vi "WPI_DashboardSeparate Tagged UDP Data.vi"(11 "String":string) -> (3 "Tagged Array":cluster{u8, u8, "unsigned byte array":u8[]}[](array[cluster]))   [LabVIEW 2017]
panel:
  out "size(s)":i32
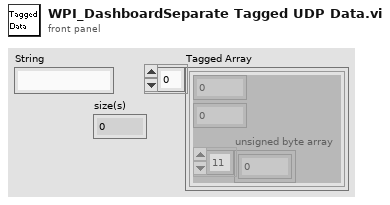
[diagram p1: front panel]
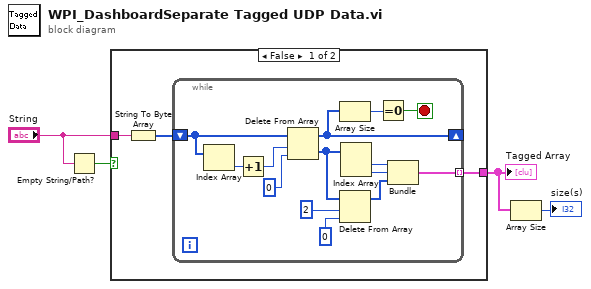
[diagram p0: block diagram]
diagram:
  n1 = Empty String/Path?(string/path="String") -> (empty?=w3:bool)
  n2 = case shown="False" w3 {
    tunnel: "String" -> [w7 _]
    tunnel: [w5 _] -> w2
    frame False {
      n3 = String To Byte Array(string=w7) -> (unsigned byte array=w6:u8[])
      n4 = while {
        shift-right: [w9] -> _
        shift-left: w6 -> [w21]
        tunnel: [w8] -> w5 mode=indexing
        stop <- w11 stop-if-true
        n5 = Index Array(array=w21) -> (element=w20:u8)  [unwired: 1 in]
        n6 = Increment(x=w20) -> (x+1=w19:u8)
        n7 = Delete From Array(array=w21, length=w19, index=0) -> (deleted portion=w16:u8[], array with subset deleted=w9:u8[])
        n8 = Array Size(array=w9) -> (size(s)=w10:i32)
        n9 = Delete From Array(array=w16, length=2, index=0) -> (array with subset deleted=w12:u8[])  [unwired: 1 out]
        n10 = Index Array(array=w16) -> (element #1=w18:u8, element #2=w17:u8)  [unwired: 2 in]
        n11 = Equal To 0?(x=w10) -> (x = 0?=w11:bool)
        n12 = Bundle(w18, w17, "unsigned byte array"=w12) -> (w8:cluster{u8, u8, "unsigned byte array":u8[]})  [unwired: 1 in]
      }
    }
    frame True {
    }
  }
  "Tagged Array" <- w2
  n13 = Array Size(array=w2) -> (size(s)=→"size(s)":i32)
